vi "swin.vi"(8 "error in (no error)":errorcluster, 11 "Duck in":refnum<class "Duck.lvclass">) -> (0 "error out":errorcluster, 2 "State":string, 3 "Duck out":refnum<class "Duck.lvclass">)   [LabVIEW 2013, in "Duck.lvclass"]
uses:
  Duck.lvclass
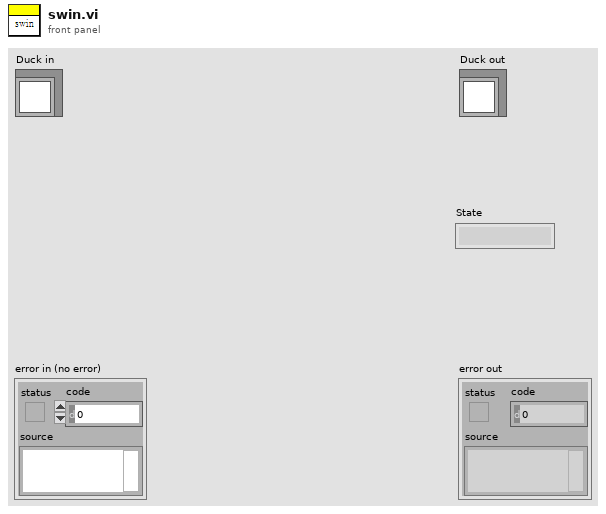
[diagram p1: front panel]
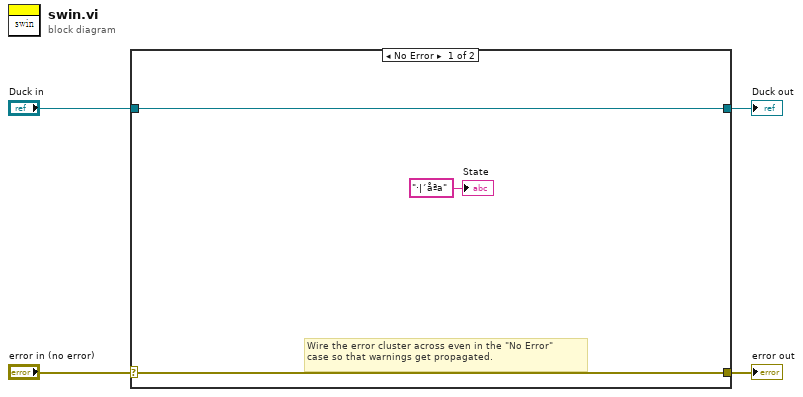
[diagram p0: block diagram]
diagram:
  n1 = case shown="No Error" "error in (no error)" {
    selector: "error in (no error)" -> [w6 w9]
    tunnel: [w6 w9] -> w3
    tunnel: [w7 w8] -> w1
    tunnel: "Duck in" -> [w7 w8]
    frame No Error {
      # "Wire the error cluster across even in the \"No Error\"\ncase so that warnings get propagated."
      "State" <- "·|´åªa" ("State")
    }
    frame Error {
    }
  }
  "error out" <- w3
  "Duck out" <- w1
